vi "Modo de Operación RC.vi"() -> ()   [LabVIEW 2013]
uses:
  <vilib>/Instr/_visa.llb/VISA Configure Serial Port (Instr).vi
panel:
  in  "Horizon":bool
  in  "Baro":bool
  in  "Desarmar":bool
  in  "Armar":bool
  in  "Control Virtual":u16(knob) caption="Horizontal Fill Slide" scale=1000.0..2000.0
  in  "START":bool
  out "Dato Leído":string
  in  "VISA resource name":refnum<visa-resource-name>
  out "Dato mandado":string
  in  "Roll":u16
  in  "Pitch":u16
  in  "Yaw":u16
  out "Throttle":u16
  in  "Stop":bool
  # "Modo de Operación RC"
  # "Dial"
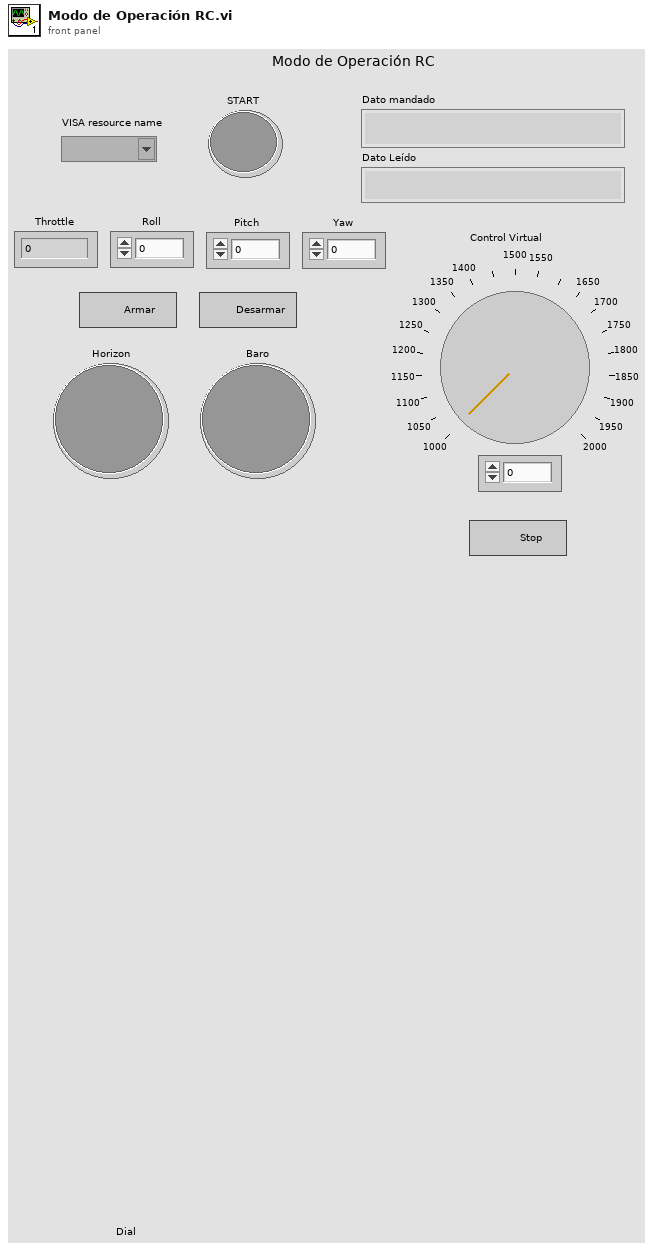
[diagram p1: front panel]
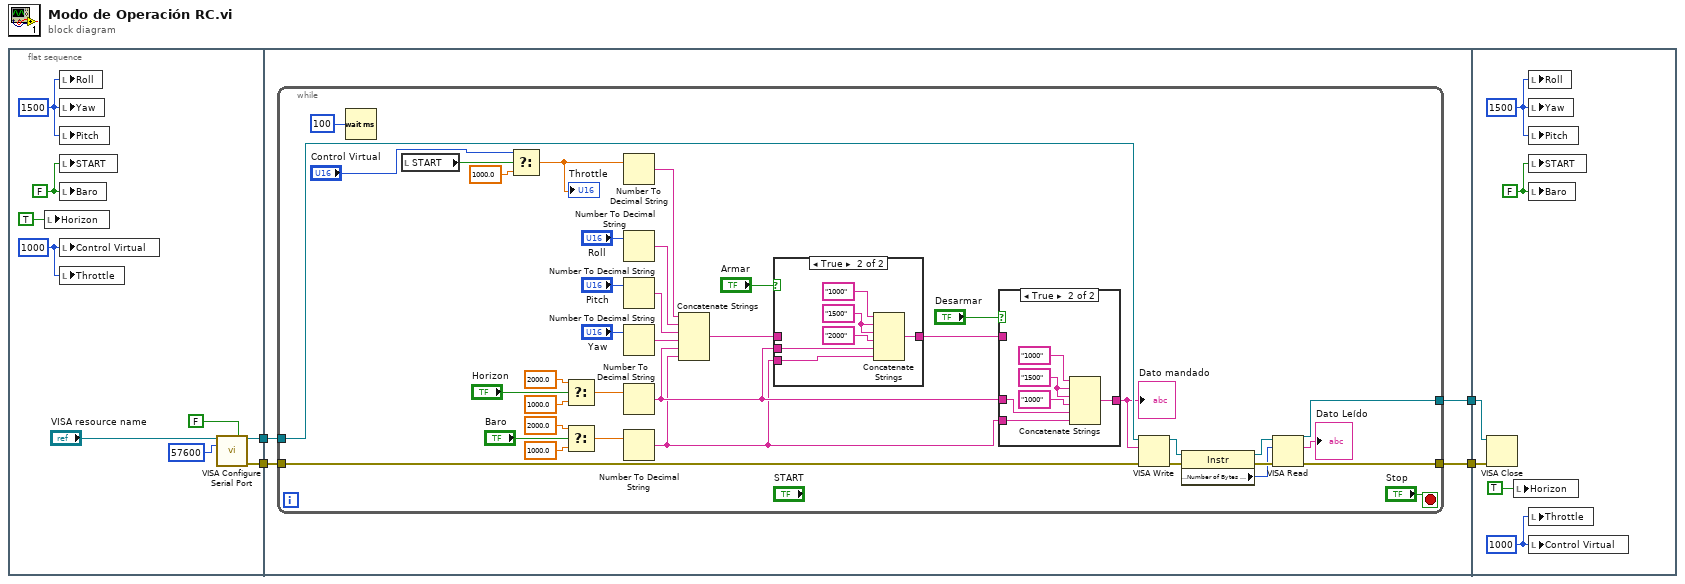
[diagram p0: block diagram]
diagram:
  n1 = flat-sequence {
    tunnel: [w10] -> w4
    tunnel: [w9] -> w3
    tunnel: w4 -> [w17]
    tunnel: w3 -> [w16]
    tunnel: [w15] -> w2
    tunnel: [w14] -> w1
    tunnel: w2 -> [w73]
    tunnel: w1 -> [w74]
    frame #0 {
      w7 = FALSE ("START")
      w6 = u16 1000
      w8 = u16 1500
      n2 = local write "Horizon"(TRUE ("Horizon")) -> ()
      n3 = local write "Roll"(w8) -> ()
      n4 = local write "Yaw"(w8) -> ()
      n5 = local write "Pitch"(w8) -> ()
      n6 = local write "START"(w7) -> ()
      n7 = local write "Baro"(w7) -> ()
      n8 = local write "Control Virtual"(w6) -> ()
      n9 = local write "Throttle"(w6) -> ()
      n10 = call-poly "VISA Configure Serial Port"("VISA resource name"="VISA resource name", "Enable Termination\nChar (T)"=FALSE ("Enable Termination\nChar (T)"), "baud rate (9600)"=u32 57600) -> ("VISA resource name out"=w10:refnum<visa-resource-name>, "error out"=w9:errorcluster)  [unwired: 11 in]
    }
    frame #1 {
      n11 = while {
        tunnel: w17 -> [w50]
        tunnel: w16 -> [w49]
        tunnel: [w43] -> w15
        tunnel: [w42] -> w14
        stop <- "Stop" stop-if-true
        n12 = Wait (ms)(milliseconds to wait=u32 100) -> ()  [unwired: 1 out]
        n13 = local read "START"() -> (w39:bool)
        n14 = Select(t="Control Virtual", s=w39, f=1000.0) -> (s? t:f=w38:dbl)
        "Throttle" <- w38
        n15 = Select(t=2000.0, s="Horizon", f=1000.0) -> (s? t:f=w18:dbl)
        n16 = Select(t=2000.0, s="Baro", f=1000.0) -> (s? t:f=w22:dbl)
        n17 = Number To Decimal String(number=w38) -> (decimal integer string=w54:string)  [unwired: 1 in]
        n18 = Number To Decimal String(number="Roll") -> (decimal integer string=w53:string)  [unwired: 1 in]
        n19 = Number To Decimal String(number="Pitch") -> (decimal integer string=w52:string)  [unwired: 1 in]
        n20 = Number To Decimal String(number="Yaw") -> (decimal integer string=w51:string)  [unwired: 1 in]
        n21 = Number To Decimal String(number=w18) -> (decimal integer string=w33:string)  [unwired: 1 in]
        n22 = Number To Decimal String(number=w22) -> (decimal integer string=w32:string)  [unwired: 1 in]
        n23 = Concatenate Strings(w54, w53, w52, w51, w33, w32) -> (w36:string)
        n24 = case shown="True" "Armar" {
          tunnel: w33 -> [_ w66]
          tunnel: w32 -> [_ w65]
          tunnel: w36 -> [w63 _]
          tunnel: [w63 w64] -> w35
          frame False {
          }
          frame True {
            w68 = "1500" ("string")
            n25 = Concatenate Strings("1000" ("string"), w68, w68, "2000" ("string"), w66, w65) -> (w64:string)
          }
        }
        n26 = case shown="True" "Desarmar" {
          tunnel: w33 -> [_ w59]
          tunnel: w32 -> [_ w58]
          tunnel: w35 -> [w56 _]
          tunnel: [w56 w57] -> w31
          frame False {
          }
          frame True {
            w61 = "1500" ("string")
            n27 = Concatenate Strings("1000" ("string"), w61, w61, "1000" ("string"), w59, w58) -> (w57:string)
          }
        }
        "Dato mandado" <- w31
        n28 = VISA Write(VISA resource name=w50, write buffer=w31, error in (no error)=w49) -> (VISA resource name out=w47:refnum<visa-resource-name>, error out=w48:errorcluster)  [unwired: 1 out]
        n29 = property class="Instr"(reference=w47, error in=w48) -> (reference out=w45:refnum<visa-resource-name>, error out=w46:errorcluster, "Serial Settings:Number of Bytes at Serial Port"=w44:u32)
        n30 = VISA Read(VISA resource name=w45, byte count=w44, error in (no error)=w46) -> (VISA resource name out=w42:refnum<visa-resource-name>, read buffer=→"Dato Leído":string, error out=w43:errorcluster)  [unwired: 1 out]
      }
    }
    frame #2 {
      w72 = FALSE ("START")
      w71 = u16 1000
      w75 = u16 1500
      n31 = VISA Close(VISA resource name=w74, error in (no error)=w73) -> ()  [unwired: 1 out]
      n32 = local write "Horizon"(TRUE ("Horizon")) -> ()
      n33 = local write "Roll"(w75) -> ()
      n34 = local write "Yaw"(w75) -> ()
      n35 = local write "Pitch"(w75) -> ()
      n36 = local write "START"(w72) -> ()
      n37 = local write "Baro"(w72) -> ()
      n38 = local write "Throttle"(w71) -> ()
      n39 = local write "Control Virtual"(w71) -> ()
    }
  }
